vi "_Set Control Values by Index.vi"(8 "error in (no error)":errorcluster, 9 "data values":variant[](array[variant]), 10 "control indexes":i32[](array[numeric]), 11 "VI Refnum":refnum<vi>) -> (0 "error out":errorcluster)   [LabVIEW 2017, in "TagDB.lvlib"]
uses:
  TagDB.lvlib
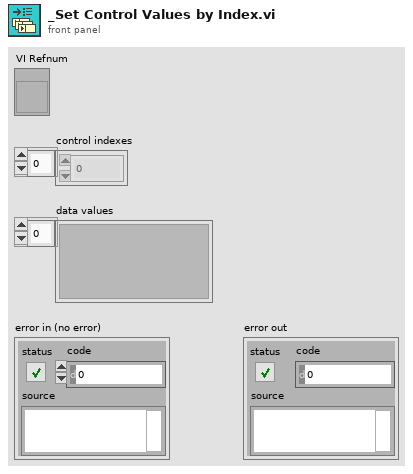
[diagram p1: front panel]
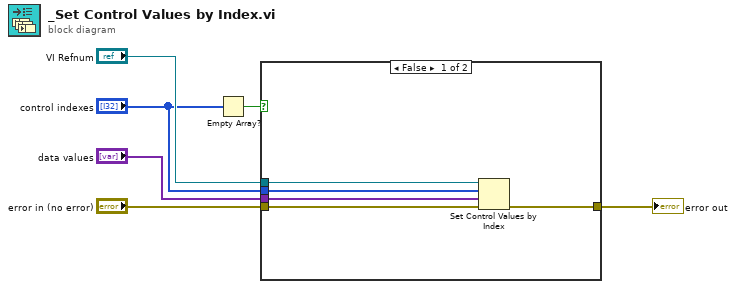
[diagram p0: block diagram]
diagram:
  n1 = Empty Array?(array="control indexes") -> (empty?=w1:bool)
  n2 = case shown="False" w1 {
    tunnel: [w11 w12] -> w6
    tunnel: "data values" -> [w10 _]
    tunnel: "error in (no error)" -> [w9 w12]
    tunnel: "VI Refnum" -> [w8 _]
    tunnel: "control indexes" -> [w7 _]
    frame False {
      n3 = Set Control Values by Index(0:w8, 1:w7, 2:w10, 3:w9) -> (11:w11:errorcluster)
    }
    frame True {
    }
  }
  "error out" <- w6
